vi "TimeSyncSrv_Exec.vi"(8 "error in (no error)":errorcluster) -> ()   [LabVIEW 2019, in "PhotonVisionLib.lvlib"]
doc: "Execute a PhotonVision Time Sync Server. It listens for UDP requests from PhotonVision devices and responds with the current FPGA time.\n\nThis VI contains a loop. Do not place this in another loop.\n\nPlace this all by itself in Periodic Tasks.\n\n\nInputs:\n -- Error In -- Optional error input cluster.\n\nOutputs:\n -- <None>"
uses:
  PhotonVisionLib.lvlib
  <vilib>/Rock Robotics/WPI/ThirdParty/JAS_Junk/TrajLib/VI/Util_GetTime_U32.vi
  PhotonVision_Globals.vi
  <vilib>/Rock Robotics/WPI/ThirdParty/JAS_Junk/TrajLib/VI/Util_GetTime_U64.vi
  <vilib>/Rock Robotics/WPI/ThirdParty/JAS_Junk/TrajLib/Trajectory_Library.lvlib
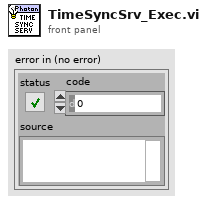
[diagram p1: front panel]
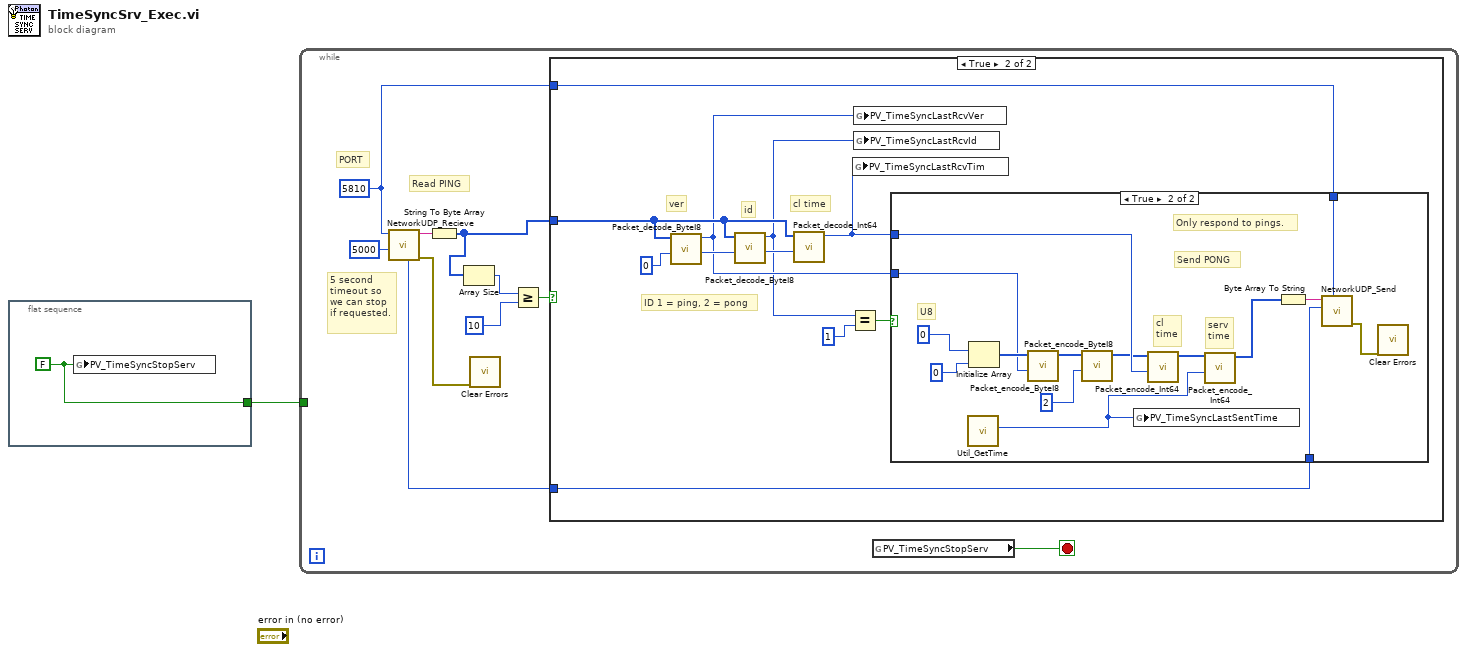
[diagram p0: block diagram]
diagram:
  n1 = flat-sequence {
    tunnel: [w2] -> w1
    frame #0 {
      w2 = FALSE ("PV_TimeSyncStopServ")
      n2 = global write "PhotonVision_Globals.vi" "PV_TimeSyncStopServ"(w2) -> ()
    }
  }
  n3 = while {
    tunnel: w1 -> [_]
    stop <- w4 stop-if-true
    w12 = u16 5810 ("receiver port")
    # "Read PING"
    # "PORT"
    # "5 second\ntimeout so\nwe can stop\nif requested."
    n4 = call <vilib>:"NetworkUDP_Recieve.vi"("timeout ms (25000)"=5000, "receiver port"=w12) -> ("error out"=w3:errorcluster, "data out"=w10:string, "SenderAddress"=w6:u32)  [unwired: 5 in, 2 out]
    n5 = String To Byte Array(string=w10) -> (unsigned byte array=w9:u8[])
    n6 = Array Size(array=w9) -> (size(s)=w8:i32)
    n7 = call <vilib>:"Clear Errors.vi"("error in (no error)"=w3) -> ()  [unwired: 5 in, 2 out]
    n8 = Greater Or Equal?(x=w8, y=10) -> (x >= y?=w11:bool)
    n9 = case shown="True" w11 {
      tunnel: w12 -> [_ w21]
      tunnel: w9 -> [_ w20]
      tunnel: w6 -> [_ w19]
      frame False {
      }
      frame True {
        # "ID 1 = ping, 2 = pong"
        # "cl time"
        # "id"
        # "ver"
        n10 = call "Packet_decode_ByteI8.vi"("StartByte"=0, "RawData"=w20) -> ("NextByte"=w22:i32, "Int8_Value"=w16:i8)  [unwired: 8 in]
        n11 = call "Packet_decode_ByteI8.vi"("StartByte"=w22, "RawData"=w20) -> ("NextByte"=w18:i32, "Int8_Value"=w14:i8)  [unwired: 8 in]
        n12 = call "Packet_decode_Int64.vi"("StartByte"=w18, "RawData"=w20) -> ("Int64_Value"=w17:i64)  [unwired: 8 in, 1 out]
        n13 = Equal?(x=w14, y=i8 1) -> (x = y?=w15:bool)
        n14 = global write "PhotonVision_Globals.vi" "PV_TimeSyncLastRcvTim"(w17) -> ()
        n15 = global write "PhotonVision_Globals.vi" "PV_TimeSyncLastRcvVer"(w16) -> ()
        n16 = global write "PhotonVision_Globals.vi" "PV_TimeSyncLastRcvId"(w14) -> ()
        n17 = case shown="True" w15 {
          tunnel: w21 -> [_ w37]
          tunnel: w19 -> [_ w30]
          tunnel: w17 -> [_ w27]
          tunnel: w16 -> [_ w24]
          frame False {
          }
          frame True {
            # "Send PONG"
            # "Only respond to pings."
            # "serv\ntime"
            # "cl\ntime"
            # "U8"
            n18 = call <vilib>:"Util_GetTime.vi"() -> ("FPGA_Time_MicroSeconds"=w29:u64)  [unwired: 9 in, 2 out]
            n19 = Initialize Array(u8 0 ("element"), 0 ("dimension size")) -> (w32:u8[])
            n20 = call "Packet_encode_ByteI8.vi"("Int8_Value"=w24, "RawData In"=w32) -> ("RawData Out"=w38:u8[])  [unwired: 9 in]
            n21 = call "Packet_encode_ByteI8.vi"("Int8_Value"=i8 2, "RawData In"=w38) -> ("RawData Out"=w26:u8[])  [unwired: 9 in]
            n22 = global write "PhotonVision_Globals.vi" "PV_TimeSyncLastSentTime"(w29) -> ()
            n23 = call "Packet_encode_Int64.vi"("Int64_Value"=w27, "RawData In"=w26) -> ("RawData Out"=w25:u8[])  [unwired: 9 in]
            n24 = call "Packet_encode_Int64.vi"("Int64_Value"=w29, "RawData In"=w25) -> ("RawData Out"=w36:u8[])  [unwired: 9 in]
            n25 = Byte Array To String(unsigned byte array=w36) -> (string=w35:string)
            n26 = call <vilib>:"NetworkUDP_Send.vi"("remote port"=w37, "IP4 Address"=w30, "data string"=w35) -> ("error out"=w28:errorcluster)  [unwired: 6 in, 2 out]
            n27 = call <vilib>:"Clear Errors.vi"("error in (no error)"=w28) -> ()  [unwired: 5 in, 2 out]
          }
        }
      }
    }
    n28 = global read "PhotonVision_Globals.vi" "PV_TimeSyncStopServ"() -> (w4:bool)
  }
